vi "Panel-FringeProcessor-2.vi"() -> ()   [LabVIEW 2009]
panel:
  out "Two outputs":i32[][](graph)
  in  "Integrate":bool
  in  "stop":bool
  out "Outputs difference":i32[](graph)
  out "X":i32
  out "Y":i32
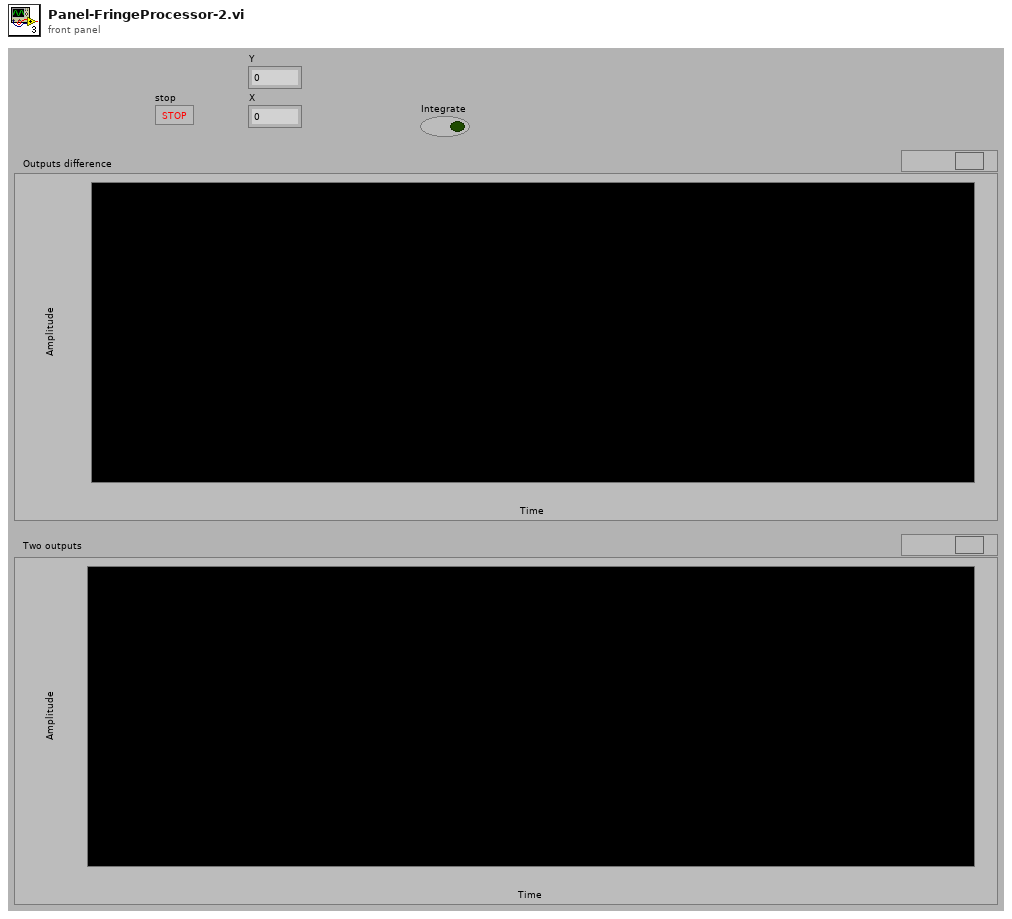
[diagram p1: front panel]
types:
  T1 = typedef "NICMOS.DATA.ctl" = cluster{"DATA":i32[][][], "INDEX":i32}
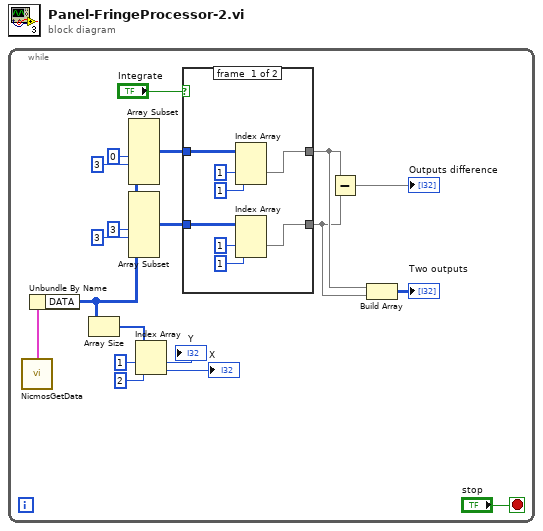
[diagram p0: block diagram]
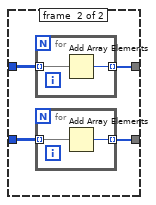
[diagram p2: hidden frame]
diagram:
  n1 = while {
    stop <- "stop" stop-if-true
    n2 = call "NicmosGetData.vi"() -> ("DATA"=w19:T1)  [unwired: 8 in, 1 out]
    n3 = Unbundle By Name(w19) -> ("DATA"=w9:i32[][][])
    n4 = Array Size(array=w9) -> (size(s)=w16:i32[])
    n5 = Array Subset(array=w9, index (dim 1)=0 ("index"), length (dim 1)=3 ("length")) -> (w8:i32[][][])  [unwired: 4 in]
    n6 = Array Subset(array=w9, index (dim 1)=3 ("index"), length (dim 1)=3 ("length")) -> (w7:i32[][][])  [unwired: 4 in]
    n7 = Index Array(array=w16, index #1=1 ("index"), index #2=2 ("index")) -> (element #1=→"Y":i32, element #2=→"X":i32)
    n8 = case shown="False" "Integrate" {
      tunnel: w8 -> [w27 w31]
      tunnel: w7 -> [w22 w30]
      tunnel: [w20 w29] -> w2
      tunnel: [w21 w28] -> w1
      frame #0 {
        n9 = Index Array(array=w27, index (dim 1)=1 ("disabled index (row)"), index (dim 2)=1 ("disabled index (col)")) -> (element=w20:i32[])  [unwired: 1 in]
        n10 = Index Array(array=w22, index (dim 1)=1 ("disabled index (row)"), index (dim 2)=1 ("disabled index (col)")) -> (element=w21:i32[])  [unwired: 1 in]
      }
      frame #1 {
        n11 = for {
          tunnel: w31 -> [w35] mode=indexing
          tunnel: [w34] -> w29 mode=indexing
          n12 = Add Array Elements(numeric array=w35) -> (sum=w34:i32)
        }
        n13 = for {
          tunnel: w30 -> [w33] mode=indexing
          tunnel: [w32] -> w28 mode=indexing
          n14 = Add Array Elements(numeric array=w33) -> (sum=w32:i32)
        }
      }
    }
    n15 = Subtract(x=w2, y=w1) -> (x-y=→"Outputs difference":i32[])
    n16 = Build Array(w2, w1) -> (→"Two outputs":i32[][])
  }
